vi "Globalna_Variabla.vi"() -> ()   [LabVIEW 2012]
panel:
  out "Direktno sa RS232":dbl[](array[numeric])
  in  "Reset":bool
  out "Sekvenca RS232":dbl[](array[numeric])
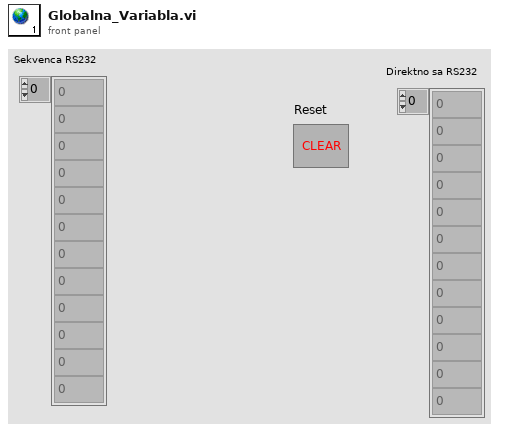
[diagram p1: front panel]
diagram:
